vi "FGV.vi"(8 "error in":errorcluster caption="entrée d'erreur") -> (0 "error out":errorcluster caption="sortie d'erreur", 3 "Local FGV":T4)   [LabVIEW 2020]
uses:
  Controls/ctrl_FGV_state.ctl
  Controls/ctrl_data_ini.ctl
  Controls/ctrl_ref_moteur.ctl
  Controls/ctrl_ref_camera.ctl
  Controls/ctrl_file_state.ctl
panel:
  in  "Data file":T1
  in  "Local FGV":T4
  in  "State_FGV":T5
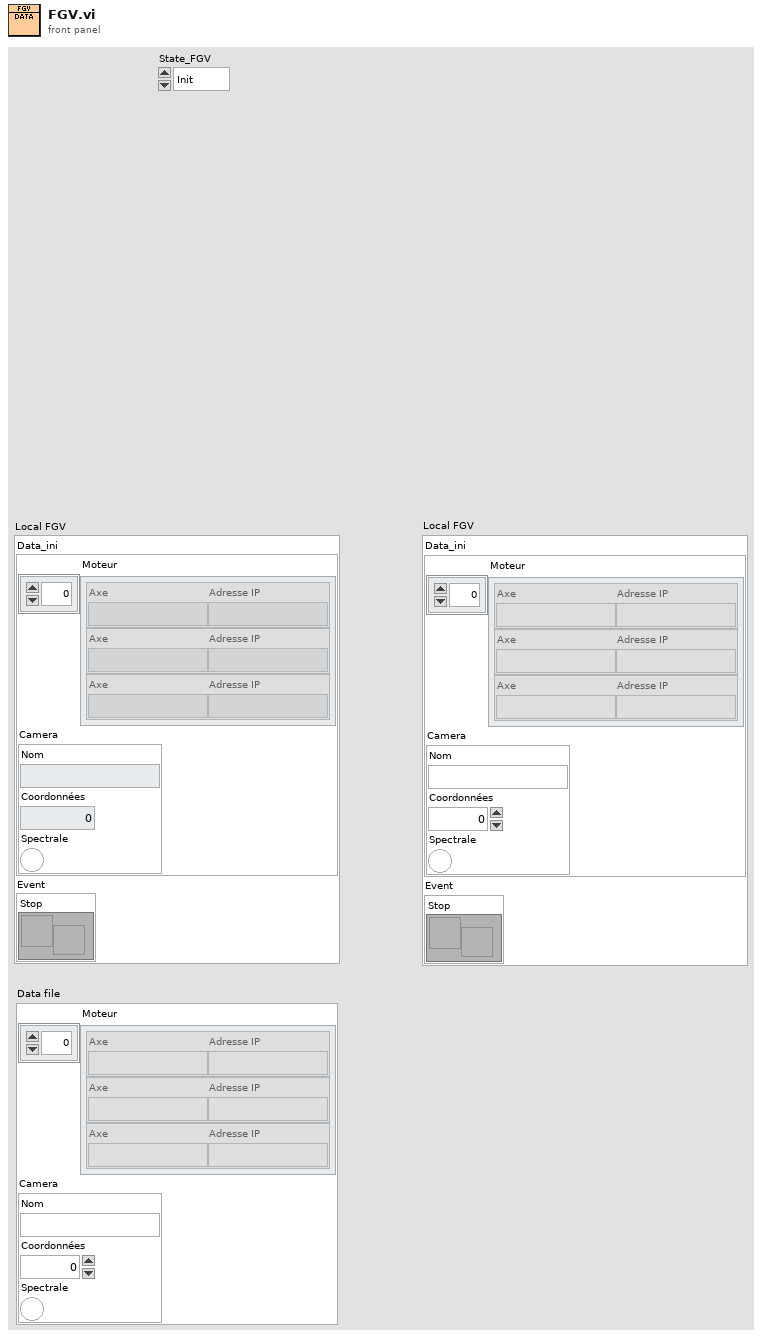
[diagram p1: front panel]
types:
  T1 = typedef "ctrl_data_ini.ctl" = cluster{"Moteur":T2[], "Camera":T3}
  T2 = typedef "ctrl_ref_moteur.ctl" = cluster{"Axe":string, "Adresse IP":string}
  T3 = typedef "ctrl_ref_camera.ctl" = cluster{"Nom":string, "Coordonnées":dbl, "Spectrale":bool}
  T4 = cluster{"Data_ini":T1, "Event":cluster{"Stop":refnum<user-event>}}
  T5 = typedef "ctrl_FGV_state.ctl" = enum16{"Init", "Read Data", "Import Datata file", "Write Data", "Write File"}
  T6 = typedef "ctrl_file_state.ctl" = enum16{"Read", "Write"}
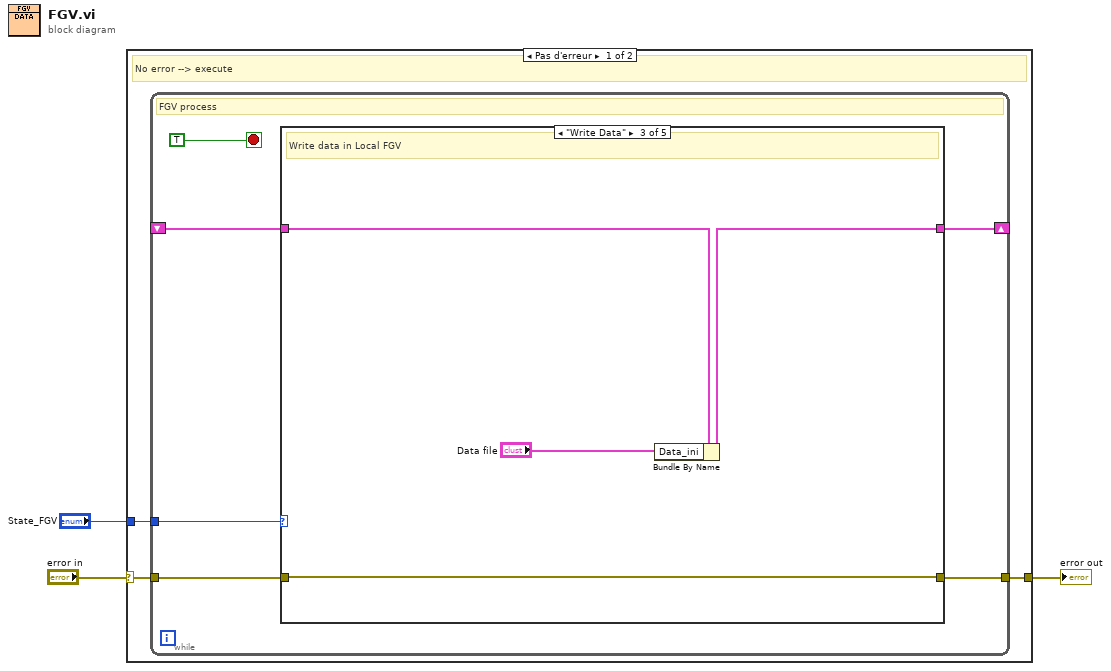
[diagram p0: block diagram]
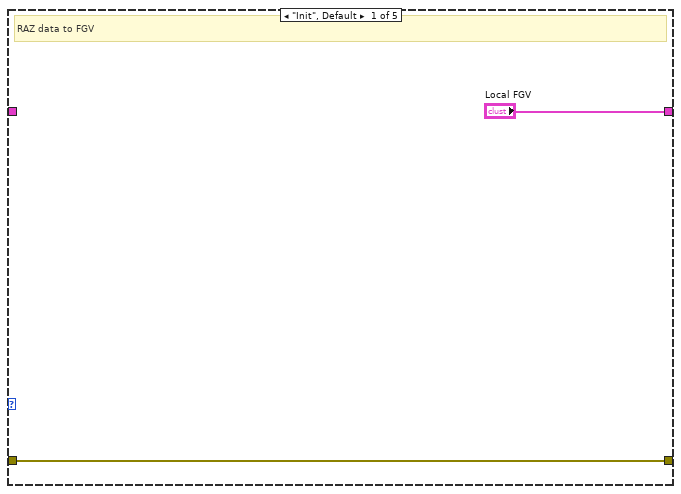
[diagram p2: hidden frame]
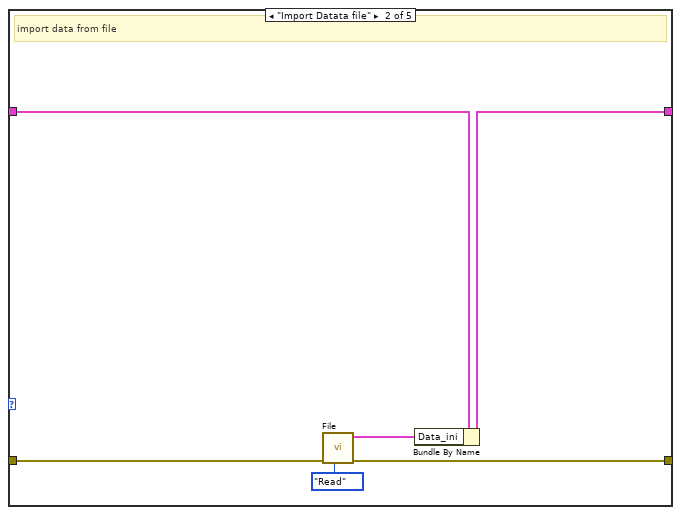
[diagram p3: hidden frame]
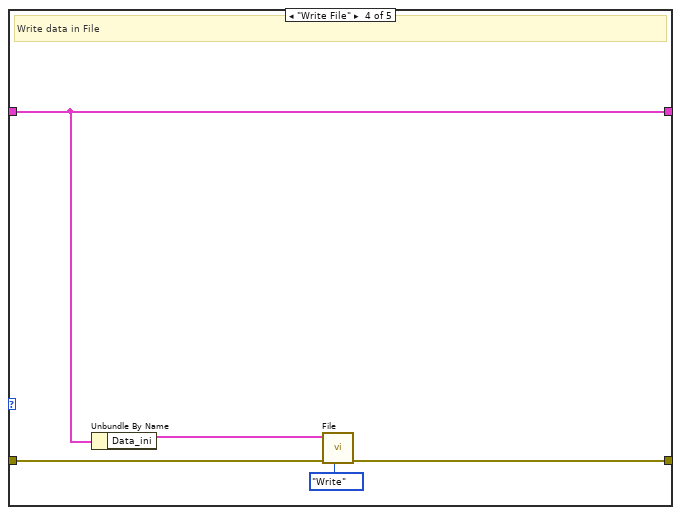
[diagram p4: hidden frame]
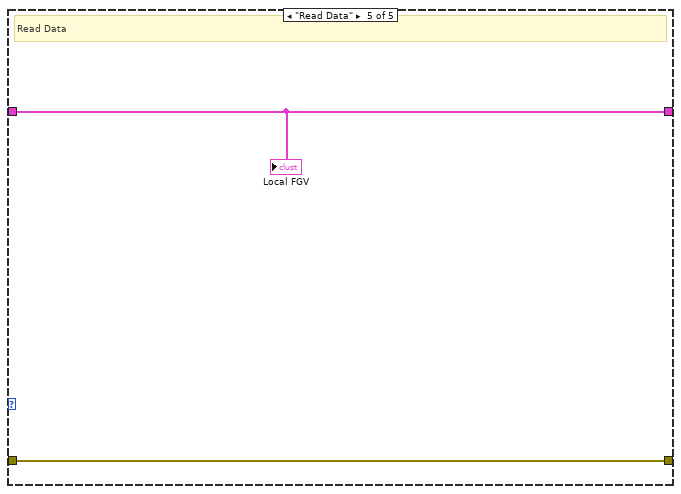
[diagram p5: hidden frame]
diagram:
  n1 = case shown="Pas d'erreur" "error in" {
    selector: "error in" -> [w5 w32]
    tunnel: [w4 w32] -> w2
    tunnel: "State_FGV" -> [w6 _]
    frame No Error {
      # "No error --> execute"
      n2 = while {
        tunnel: w6 -> [w7]
        tunnel: w5 -> [w12]
        tunnel: [w11] -> w4
        shift-right: [w9] -> _
        shift-left: _ -> [w8]
        stop <- TRUE stop-if-true
        # "FGV process"
        n3 = case shown="\"Write Data\"" w7 {
          tunnel: w12 -> [w14 w20 w24 w29 w30]
          tunnel: [w14 w19 w24 w28 w30] -> w11
          tunnel: ["Local FGV" w16 w22 w26 w31] -> w9
          tunnel: w8 -> [_ w17 w23 w26 w31]
          frame "Init", Default {
            # "RAZ data to FGV"
          }
          frame "Import Datata file" {
            # "import data from file"
            n4 = call "File.vi"("File_state"=ctrl_file_state."Read", "error in"=w20) -> ("error out"=w19:errorcluster, "Data_ini_Write"=w15:T1)  [unwired: 8 in]
            n5 = Bundle By Name(cluster=w17, "Data_ini"=w15) -> (w16:T4)
          }
          frame "Write Data" {
            # "Write data in Local FGV"
            n6 = Bundle By Name(cluster=w23, "Data_ini"="Data file") -> (w22:T4)
          }
          frame "Write File" {
            # "Write data in File"
            n7 = Unbundle By Name(w26) -> ("Data_ini"=w25:T1)
            n8 = call "File.vi"("File_state"=ctrl_file_state."Write", "error in"=w29, "Data_ini_Read"=w25) -> ("error out"=w28:errorcluster)  [unwired: 7 in, 1 out]
          }
          frame "Read Data" {
            # "Read Data"
            "Local FGV" <- w31
          }
        }
      }
    }
    frame Error {
      # "Error --> no execution"
    }
  }
  "error out" <- w2
